vi "lv_icon.vi"(6 "error in (no error)":errorcluster, 7 "VI REF In":refnum<vi>, 8 "From Editor":bool=TRUE, 10 "Color icon in":T8, 11 "BW icon in":T8) -> (0 "Error code out":i32, 2 "Color icon out":T8, 3 "BW icon out":T8, 4 "error out":errorcluster, 5 "VI REF Out":refnum<vi>)   [LabVIEW 2009]
doc: "Version 2.2"
uses:
  <vilib>/picture/picture.llb/imagedata.ctl
  lv_icon_SubVis/Controls/Enum/ENUM_Icon Fixer Commands.ctl
  lv_icon_SubVis/Controls/Enum/ENUM_Graphic Template select.ctl
  lv_icon_SubVis/Controls/Cluster/CLuster_Line Fit Results.ctl
  lv_icon_SubVis/Controls/Enum/ENUM RB_Fit Result.ctl
  lv_icon_SubVis/Controls/String_Picture/Picture_Icon.ctl
  lv_icon_SubVis/Controls/Enum/ENUM_Icon Sizing.ctl
  lv_icon_SubVis/Controls/Enum/RBENUM_Icon Position.ctl
  lv_icon_SubVis/Controls/Cluster/Cluster_Icon Fixer Command Data Set.ctl
  lv_icon_SubVis/Controls/Enum/ENUM_Clear Text Select.ctl
  lv_icon_SubVis/Controls/Enum/ENUM_Set Focus Select.ctl
  lv_icon_SubVis/Controls/Enum/ENUM_Frame Template Select.ctl
  lv_icon_SubVis/Controls/Array/String Array_Body Text.ctl
  lv_icon_SubVis/Controls/String_Picture/STRING_Line Display.ctl
  <vilib>/event_ctls.llb/eventvkey.ctl
  lv_icon_SubVis/Controls/Cluster/Cluster_Sizing Data.ctl
panel:
  in  "stop Keys":bool
  in  "Position":T1=enum."MID-CTR"
  in  "Rule":T2
  in  "Header":bool=TRUE
  in  "Rows":u32=5 min=1 max=5 step=1
  in  "Width":u32=32 min=7 max=32 step=1
  in  "Default sizing":bool
  in  "Random Colors":bool
  out "stop draw":bool
  in  "Reset to Old":bool
  in  "Clear All text":bool
  out "Old":T3 caption="Icon"
  in  "Exit Use Old":bool
  out "New":T3 caption="Icon"
  in  "Exit Use New":bool
  out "History":T3[](array[typedef])
  in  "Frame Select":enum32{"2 Color", "5 Color"}(tab)
  out "Secondary":u32(colorbox)=16448250
  out "Primary":u32(colorbox)=239
  out "Body Back":u32(colorbox)=16448250 caption="Back"
  out "Body txt":u32(colorbox) caption="Text"
  out "Frame":u32(colorbox)
  out "Header txt":u32(colorbox)=65793 caption="Text"
  out "Header Back":u32(colorbox)=239 caption="Back"
  in  "NI Editor":bool
  in  "Close Vi Ref":bool
  out "VI Name":string
  in  "Line 4":string
  in  "Line 3":string
  in  "Line 2":string
  in  "Line 1":string
  in  "Header":string
  out "Data Array":T4[](array[typedef])
  in  "Select Graphic In":T6
  out "Cmd":T7=enum."Initialize"
  out "Big ICON":picture caption="Icon"
  out "timed out?":bool
  # "Icon Sizing"
  # "History"
  # "Make your own icon editor..."
  # "Use this template to create your own icon editor that replaces the built-in LV icon editor. To do so, you must save your new editor as \"lv_icon.vi\" in the same plugins directory where this template resides. Thereafter, whenever you edit an icon in LabVIEW, this VI will execute in place of the LV icon editor. \n\nThe VI's current black/white and color icons are passed as inputs. Your editor should output the modified black/white and color icons and an error code. If you output any non-zero error code, the VI's icons will not be modified. Error code 43 (cancelError) will simply leave the icon unchanged. All other error codes will cause LV's built-in icon editor to launch. This is useful in case there's a bug in your plug-in icon editor.\n\nDo not change connector pane. Do not change the names of any of the  controls or indicators connected to the conpane. You may hide any or all of these controls and add whatever interface you desire. You may decide to call a third party graphics editing tool and leverage that tool for editing your icons in LV."
  # "Body Back\nHeader Text"
  # "Frame\nBody Text\nHeader Back"
  # "Body"
  # "Header"
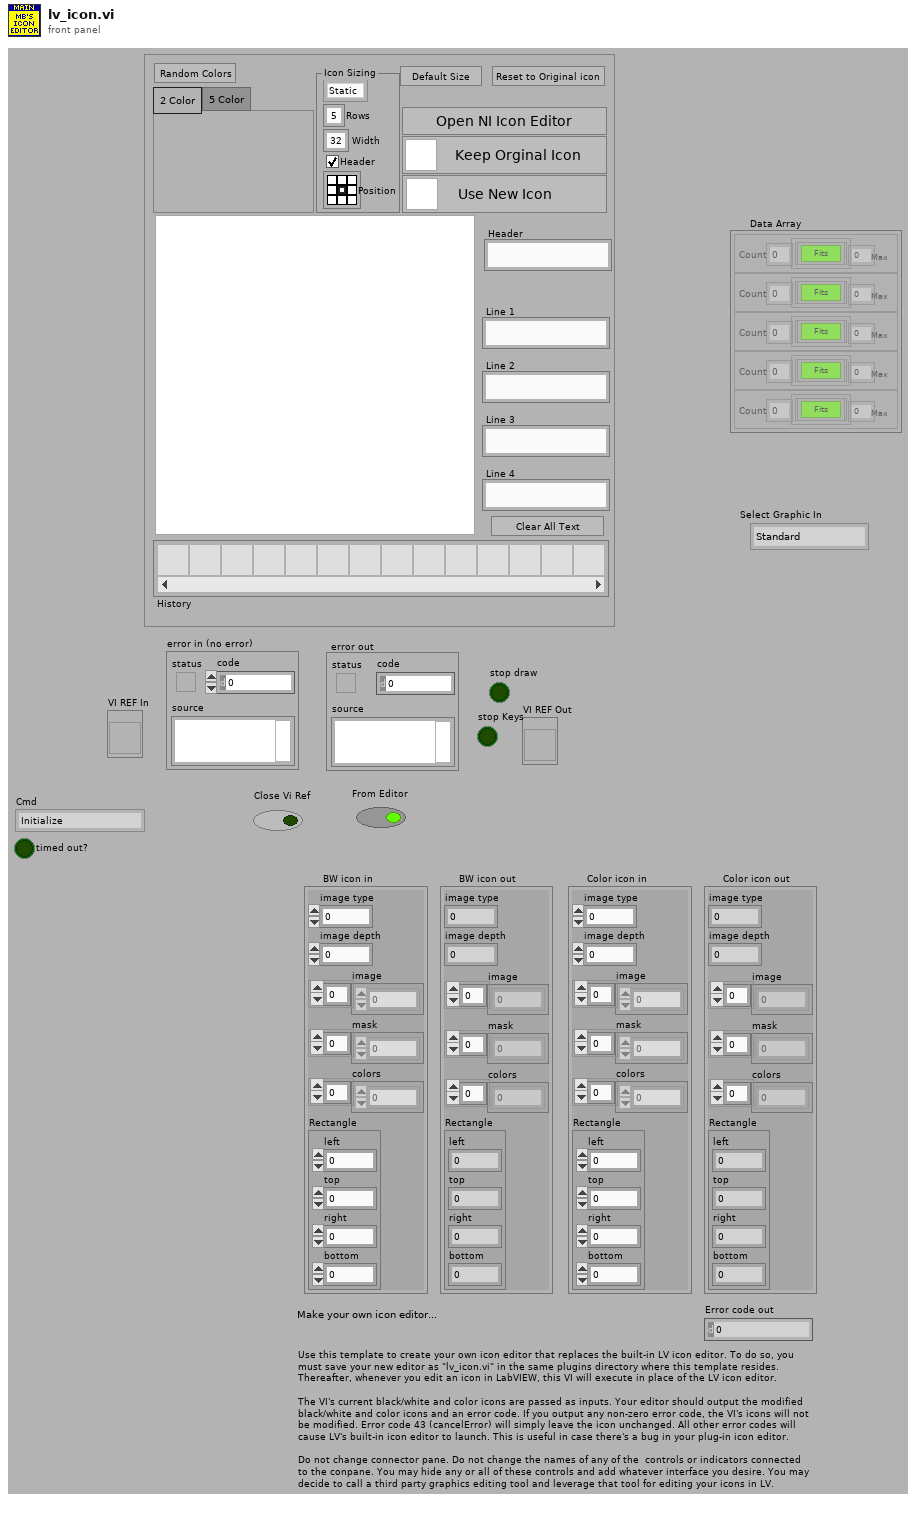
[diagram p1: front panel]
types:
  T1 = typedef "RBENUM_Icon Position.ctl" = enum32{"LFT-TOP", "MID-TOP", "RGT-TOP", "LFT-CTR", "MID-CTR", "RGT-CTR", "LFT-BOT", "MID-BOT", "RGT-BOT"}
  T2 = typedef "ENUM_Icon Sizing.ctl" = enum16{"Static", "Auto"}
  T3 = typedef "Picture_Icon.ctl" = picture
  T4 = typedef "CLuster_Line Fit Results.ctl" = cluster{"Fit Result":T5, "Max":i32, "Count":i32}
  T5 = typedef "ENUM RB_Fit Result.ctl" = enum32{"Fits", "Almost Fits", "NO Fit"}
  T6 = typedef "ENUM_Graphic Template select.ctl" = enum16{"Standard", "Standard Read", "Standard Change", "Auto Test Template"}
  T7 = typedef "ENUM_Icon Fixer Commands.ctl" = enum16{"NoNe", "Initialize", "Get VI", "Extract Icon", "ReDraw New Icon", "Set Vis Icon", "Save Vi", "Clear String controls", "Set Icon Cluster", "Reset Vis Icon", "Pick Colors", "Upload icon templates", "Download icon templates", "Stop Program", "OCR", "Display Set", "Set Focus", "Set Colors"}
  T8 = typedef "imagedata.ctl" = cluster{"image type":i32, "image depth":i32, "image":u8[], "mask":u8[], "colors":u32[], "Rectangle":cluster{"left":i16, "top":i16, "right":i16, "bottom":i16}}
  T9 = typedef "ENUM_Set Focus Select.ctl" = enum16{"NoNe", "Header", "Line 1", "Line 2", "Line 3", "Line 4", "Next", "Back"}
  T10 = typedef "ENUM_Clear Text Select.ctl" = enum16{"NoNe", "All", "Header", "Body"}
  T11 = enum32{"Invalid", "Standard", "Closed", "Hidden", "Minimized", "Maximized"}
  T12 = typedef "Cluster_Icon Fixer Command Data Set.ctl" = cluster{"Cmd":T7, "Data":variant}
  T13 = typedef "Cluster_Icon Data.ctl" = cluster{"Header":T14, "Body":T15, "ImageData":T16, "New Icon":T3, "Line Status":bool[], "Format":T18}
  T14 = typedef "STRING_Line Display.ctl" = string
  T15 = typedef "String Array_Body Text.ctl" = T14[]
  T16 = typedef "Cluster_Image Data.ctl" = cluster{"image type":i32, "image depth":i32, "image":u8[], "mask":u8[], "colors":u32[], "Rectangle":T17}
  T17 = typedef "CLuster_Selectoin Box.ctl" = cluster{"left":i16, "top":i16, "right":i16, "bottom":i16}
  T18 = typedef "Cluster_Icon Format.ctl" = cluster{"Color":T19, "Icon Sizing":T21}
  T19 = typedef "Cluster_Icon Color Set.ctl" = cluster{"Body txt":u32, "Body Back":u32, "Frame":u32, "Header txt":u32, "Header Back":u32, "type":T20}
  T20 = typedef "ENUM_Frame Template Select.ctl" = enum16{"2 Color", "5 Color"}
  T21 = typedef "Cluster_Sizing Data.ctl" = cluster{"Rule":T2, "Header":bool, "Rows":u32, "Width":u32, "Position":T1}
  T22 = typedef "eventvkey.ctl" = enum16{"ASCII", "Enter", "Return", "Shift", "Ctrl", "Alt", "Cmd", "Opt", "Caps", "NumLock", "Clear", "Break", "Up", "Down", "Left", "Right", "Insert", "Delete", "Home", "End", "PageUp", "PageDown", "Escape", "Help", "Pause", "ScrollLock", "F1", "F2", "F3", "F4", "F5", "F6", "F7", "F8", "F9", "F10", "F11", "F12", "F13", "F14", "F15", "F16", "F17", "F18", "F19", "F20", "F21", "F22", "F23", "F24", "Play", "VolumeUp", "VolumeDown", "Mute", "Two Byte Char"}
  T23 = typedef "LVRectTypeDef.ctl" = cluster{"left":i16, "top":i16, "right":i16, "bottom":i16}
  T24 = typedef "LVPoint32TypeDef.ctl" = cluster{"Horizontal":i32, "Vertical":i32}
  T25 = typedef "Bool_Otagon Stop Button no latch.ctl" = bool
  T26 = cluster{"Selection Start":u32, "Selection End":u32}
  T27 = cluster{"Rule":T2, "Header":bool, "Rows":u32, "Width":u32, "Position":T1}
  T28 = typedef "Cluster_Format Storage.ctl" = cluster{"Header":T14, "Format":T18}
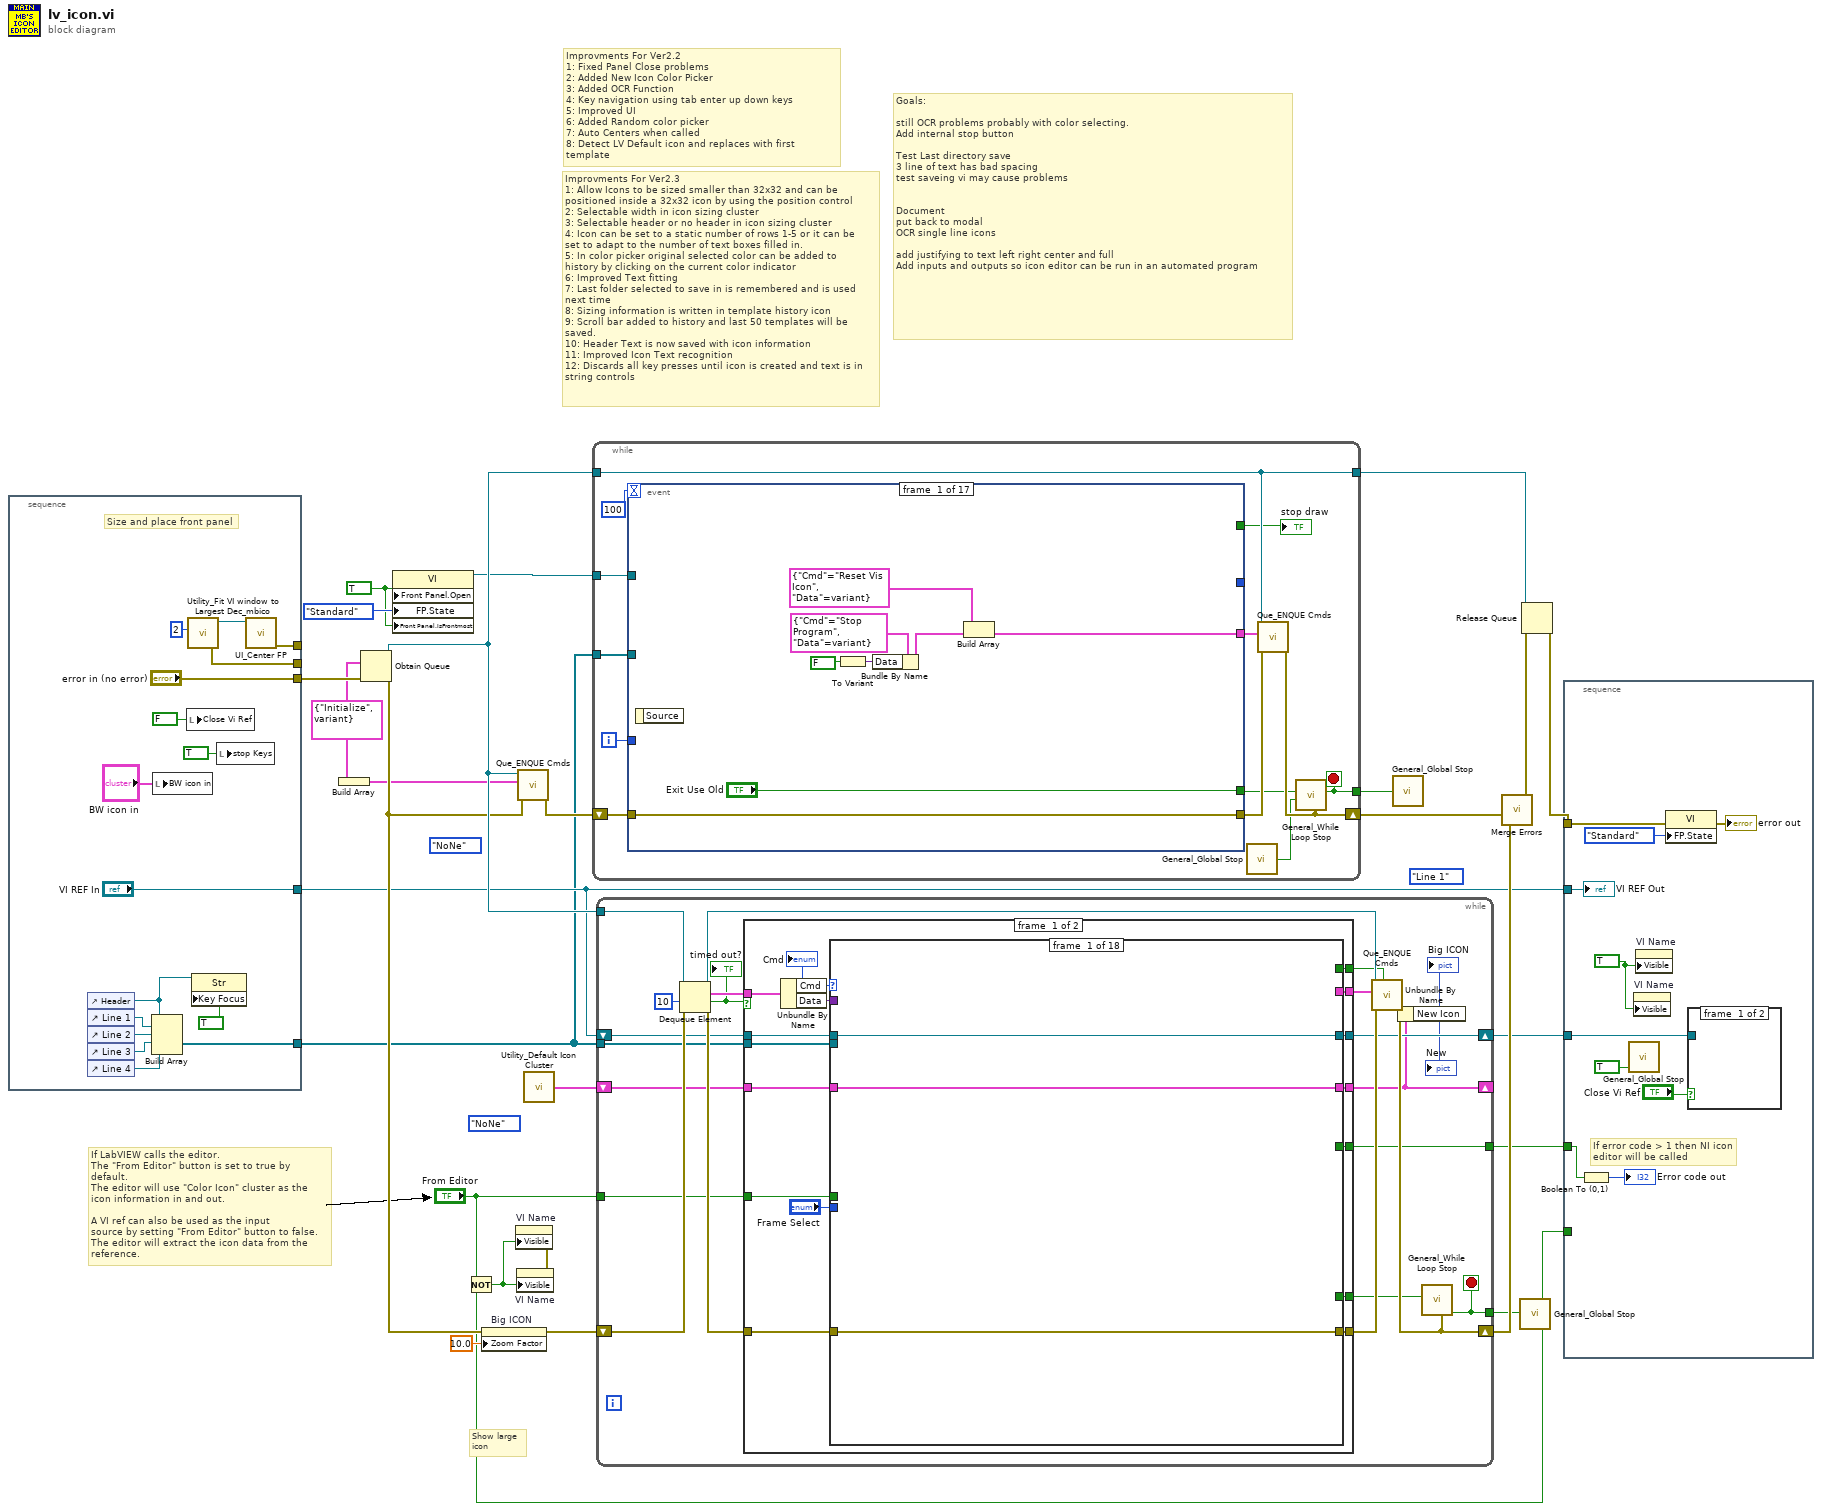
[diagram p0: block diagram]
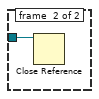
[diagram p2: hidden frame]
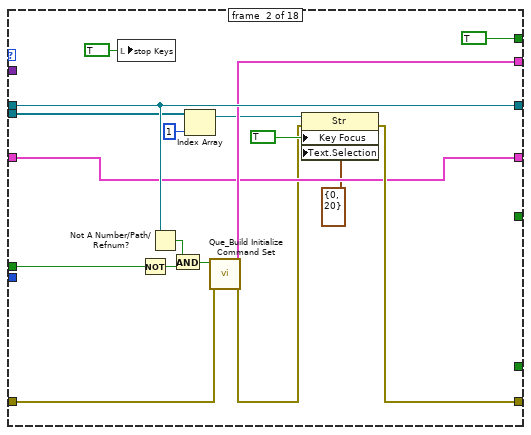
[diagram p3: hidden frame]
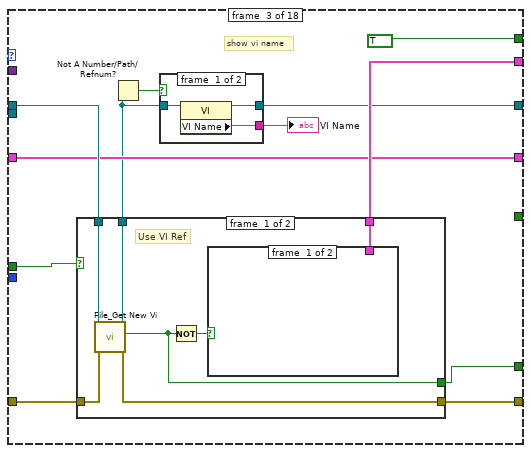
[diagram p4: hidden frame]
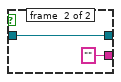
[diagram p5: hidden frame]
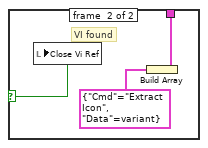
[diagram p6: hidden frame]
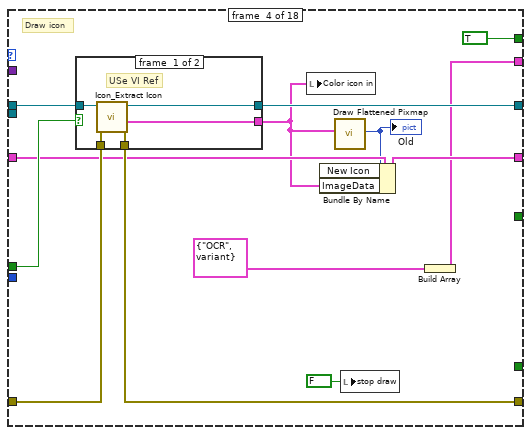
[diagram p8: hidden frame]
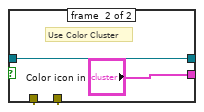
[diagram p9: hidden frame]
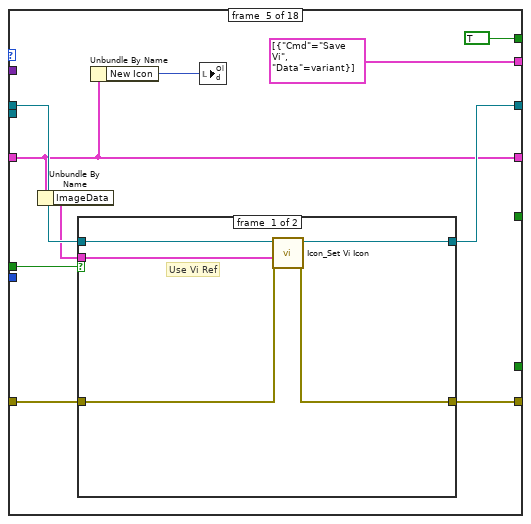
[diagram p10: hidden frame]
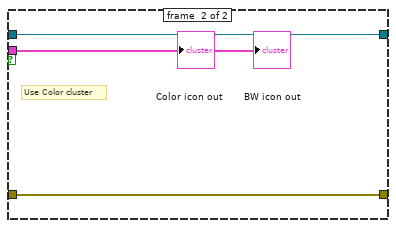
[diagram p11: hidden frame]
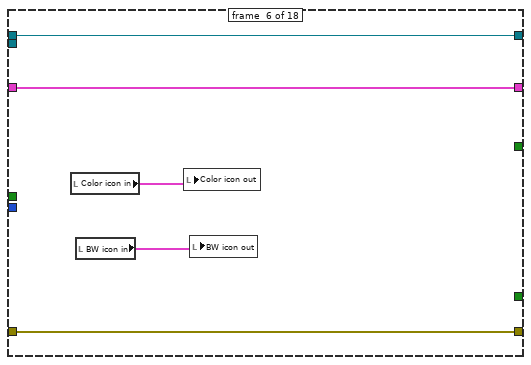
[diagram p12: hidden frame]
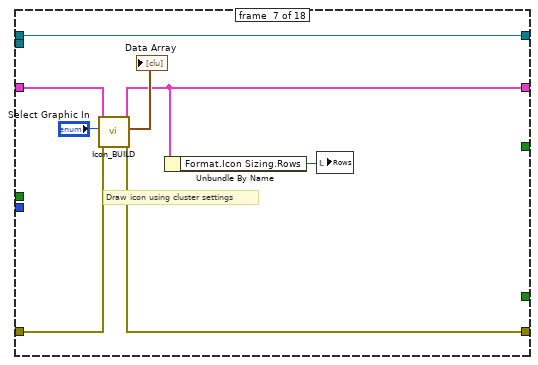
[diagram p13: hidden frame]
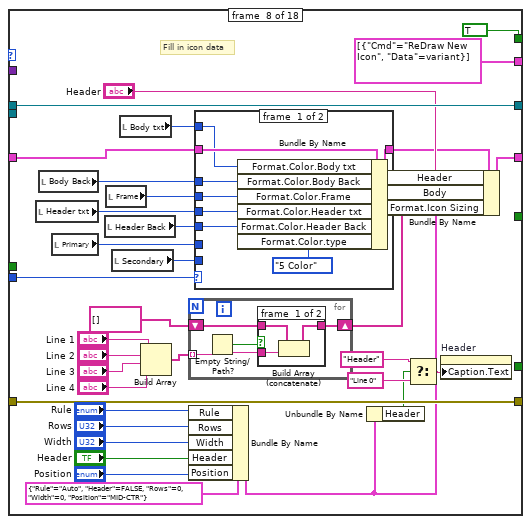
[diagram p14: hidden frame]
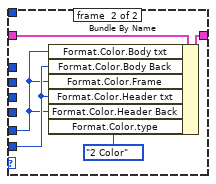
[diagram p16: hidden frame]
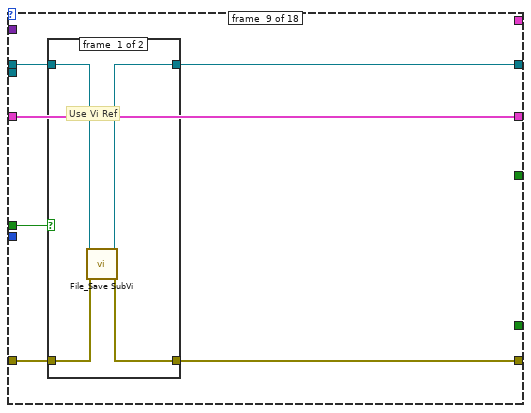
[diagram p17: hidden frame]
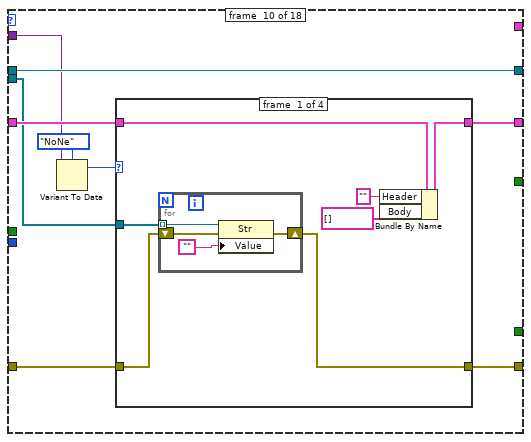
[diagram p19: hidden frame]
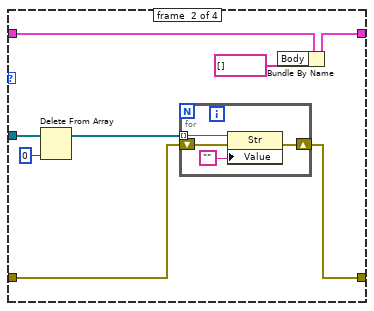
[diagram p20: hidden frame]
diagram:
  (unwired) ENUM_Set_Focus_Select."NoNe" ("Focus Select")
  (unwired) ENUM_Set_Focus_Select."Line 1" ("t")
  (unwired) ENUM_Clear_Text_Select."NoNe" ("Clear Text Select")
  w6 = TRUE ("Front Panel Window:Open")
  w12 = T12 {"Cmd"=enum."Initialize", "Data"=variant} ("Cluster")
  # "Improvments For Ver2.2\n1: Fixed Panel Close problems\n2: Added New Icon Color Picker\n3: Added OCR Function\n4: Key navigation using tab enter up down keys\n5: Improved UI \n6: Added Random color picker\n7: Auto Centers when called\n8: Detect LV Default icon and replaces with first template"
  # "Goals:\n\nstill OCR problems probably with color selecting.\nAdd internal stop button\n\nTest Last directory save\n3 line of text has bad spacing\ntest saveing vi may cause problems\n\n\nDocument\nput back to modal\nOCR single line icons\n \nadd justifying to text left right center and full\nAdd inputs and outputs so icon editor can be run in an automated program"
  # "Improvments For Ver2.3\n1: Allow Icons to be sized smaller than 32x32 and can be \npositioned inside a 32x32 icon by using the position control\n2: Selectable width in icon sizing cluster\n3: Selectable header or no header in icon sizing cluster\n4: Icon can be set to a static number of rows 1-5 or it can be\nset to adapt to the number of text boxes filled in.\n5: In color picker original selected color can be added to \nhistory by clicking on the current color indicator\n6: Improved Text fitting\n7: Last folder selected to save in is remembered and is used \nnext time\n8: Sizing information is written in template history icon\n9: Scroll bar added to history and last 50 templates will be saved.\n10: Header Text is now saved with icon information\n11: Improved Icon Text recognition\n12: Discards all key presses until icon is created and text is in \nstring controls"
  # "Show large\nicon"
  # "If LabVIEW calls the editor.\nThe \"From Editor\" button is set to true by default.\nThe editor will use \"Color Icon\" cluster as the \nicon information in and out.\n\nA VI ref can also be used as the input \nsource by setting \"From Editor\" button to false.\nThe editor will extract the icon data from the \nreference."
  n1 = stacked-sequence {
    tunnel: ["error in (no error)"] -> w22
    tunnel: ["VI REF In"] -> w10
    tunnel: [w37] -> w1
    tunnel: [w28] -> _
    tunnel: [w27] -> _
    frame #0 {
      # "Size and place front panel"
      n2 = control-ref of="Header"() -> (w35:refnum<vi>)
      n3 = control-ref of="Line 1"() -> (w38:refnum<vi>)
      n4 = control-ref of="Line 2"() -> (w39:refnum<vi>)
      n5 = control-ref of="Line 3"() -> (w40:refnum<vi>)
      n6 = control-ref of="Line 4"() -> (w41:refnum<vi>)
      n7 = Build Array(w35, w38, w39, w40, w41) -> (w37:refnum<vi>[])
      n8 = local write "BW icon in"("BW icon in") -> ()
      n9 = local write "Close Vi Ref"(FALSE ("Close Vi Ref")) -> ()
      n10 = call "Utility_Fit VI window to Largest Dec_mbico.vi"("border spacing (2 px)"=2) -> ("error out"=w28:errorcluster, "dup VI Ref"=w32:refnum<vi>)  [unwired: 5 in]
      n11 = property class="Str"(reference=w35, "Key Focus"=TRUE) -> ()  [unwired: 1 in, 2 out]
      n12 = local write "stop Keys"(TRUE ("stop Keys")) -> ()
      n13 = call "UI_Center FP.vi"("VI Ref"=w32) -> ("Error Out"=w27:errorcluster)  [unwired: 9 in, 1 out]
    }
  }
  n14 = Build Array(w12) -> (w11:T12[])
  n15 = Obtain Queue(element data type=w12, error in (no error)=w22) -> (queue out=w21:refnum<queue>, error out=w16:errorcluster)  [unwired: 3 in, 1 out]
  n16 = property class="VI"("Front Panel.Open"=w6, "FP.State"=T11."Standard" ("Front Panel Window:State"), "Front Panel.IsFrontmost"=w6) -> (reference out=w14:refnum<vi>)  [unwired: 2 in, 1 out]
  n17 = Not(x="From Editor") -> (.not. x?=w2:bool)
  n18 = property on="Big ICON" class="Picture"(error in=w16, "Zoom Factor"=sgl 10.0) -> (error out=w15:errorcluster)  [unwired: 1 in, 1 out]
  n19 = property on="VI Name" class="Str"("Visible"=w2) -> (error out=w3:errorcluster)  [unwired: 2 in, 1 out]
  n20 = property on="VI Name" class="Str"(error in=w3, "Visible"=w2) -> ()  [unwired: 1 in, 2 out]
  n21 = call "Que_ENQUE Cmds.vi"("Error"=w16, "Array"=w11, "Queue Ref"=w21) -> ("Error Out"=w20:errorcluster)  [unwired: 8 in]
  n22 = call "Utility_Default Icon Cluster.vi"() -> ("Default Cluster"=w13:T13)  [unwired: 2 in]
  n23 = while {
    shift-right: [w52] -> w25
    shift-left: w20 -> [w48]
    tunnel: w21 -> [w49]
    tunnel: [w49] -> w26
    tunnel: [w50] -> w9
    tunnel: w14 -> [w47]
    tunnel: w1 -> [w43]
    i -> [w45]
    stop <- w50 stop-if-true
    n24 = event shown="[4] \"NI Editor\": Value Change" {
      selector: _ -> [_ _ _ _ _ _ _ _ _ _ _ _ _ _ _ _ _]
      dyn-events: _ -> [_ _ _ _ _ _ _ _ _ _ _ _ _ _ _ _ _]
      timeout: 100 -> [_ _ _ _ _ _ _ _ _ _ _ _ _ _ _ _ _]
      tunnel: w48 -> [w63 w65 w71 w81 w89 w98 w99 w109 w129 w141 w148 w155 w193 w211 w213 w215 w217]
      tunnel: [w63 w65 w71 w81 w89 w98 w99 w110 w129 w133 w148 w154 w192 w211 w213 w215 w217] -> w54
      tunnel: ["Exit Use Old" _ _ "Exit Use New" "NI Editor" TRUE _ _ _ _ _ _ _ _ _ _ _] -> w51
      tunnel: [w62 w66 T12[] [{"Cmd"=enum."Initialize", "Data"=variant}] w80 w88 w90 w101 w107 _ w140 T12[] [{"Cmd"=enum."Set Icon Cluster", "Data"=variant}] w152 w191 T12[] [{"Cmd"=enum."Set Icon Cluster", "Data"=variant}] T12[] [{"Cmd"=enum."ReDraw New Icon", "Data"=variant}] T12[] [{"Cmd"=enum."Set Icon Cluster", "Data"=variant}] w219] -> w53
      tunnel: w47 -> [_ _ _ _ _ _ _ w117 w128 _ _ _ _ _ _ _ _]
      tunnel: w45 -> [_ _ _ _ _ _ _ _ w127 _ _ _ _ _ _ _ _]
      tunnel: [_ _ _ _ _ _ _ _ w124 _ _ _ _ _ _ _ _] -> w44
      tunnel: w43 -> [_ _ _ _ _ _ _ _ _ _ _ w151 w189 _ _ _ _]
      tunnel: [_ _ _ _ _ _ _ _ _ w136 _ _ _ _ _ _ _] -> _
      event #0 {
        n25 = event-data() -> ()  [unwired: 1 in, 1 out]
        n26 = To Variant(anything=FALSE) -> (Variant=w59:variant)
        n27 = Bundle By Name(cluster=T12 {"Cmd"=enum."Stop Program", "Data"=variant} ("element"), "Data"=w59) -> (w60:T12)
        n28 = Build Array(T12 {"Cmd"=enum."Reset Vis Icon", "Data"=variant} ("element"), w60) -> (w62:T12[])
      }
      event #1 {
        n29 = event-data() -> ()  [unwired: 1 in, 1 out]
        n30 = To Variant(anything=ENUM_Clear_Text_Select."All" ("Clear Text Select")) -> (Variant=w67:variant)
        n31 = Bundle By Name(cluster=T12 {"Cmd"=enum."Clear String controls", "Data"=variant} ("Cluster"), "Data"=w67) -> (w69:T12)
        n32 = Build Array(w69, T12 {"Cmd"=enum."ReDraw New Icon", "Data"=variant} ("element")) -> (w66:T12[])
      }
      event #2 {
        n33 = event-data() -> ()  [unwired: 1 in, 1 out]
      }
      event #3 {
        n34 = event-data() -> ()  [unwired: 1 in, 1 out]
        n35 = To Variant(anything=FALSE) -> (Variant=w77:variant)
        n36 = Bundle By Name(cluster=T12 {"Cmd"=enum."Stop Program", "Data"=variant} ("element"), "Data"=w77) -> (w78:T12)
        n37 = Build Array(T12 {"Cmd"=enum."Download icon templates", "Data"=variant} ("element"), T12 {"Cmd"=enum."Set Vis Icon", "Data"=variant} ("element"), w78) -> (w80:T12[])
      }
      event #4 {
        n38 = event-data() -> ()  [unwired: 1 in, 1 out]
        n39 = To Variant(anything=TRUE) -> (Variant=w85:variant)
        n40 = Bundle By Name(cluster=T12 {"Cmd"=enum."Stop Program", "Data"=variant} ("element"), "Data"=w85) -> (w86:T12)
        n41 = Build Array(T12 {"Cmd"=enum."Reset Vis Icon", "Data"=variant} ("element"), w86) -> (w88:T12[])
      }
      event #5 {
        n42 = event-data() -> ()  [unwired: 1 in, 1 out]
        n43 = To Variant(anything=TRUE) -> (Variant=w93:variant)
        n44 = Bundle By Name(cluster=T12 {"Cmd"=enum."Stop Program", "Data"=variant} ("element"), "Data"=w93) -> (w94:T12)
        n45 = Build Array(T12 {"Cmd"=enum."Reset Vis Icon", "Data"=variant} ("element"), w94) -> (w90:T12[])
        n46 = event-data("Discard?"=TRUE) -> ()  [unwired: 1 in, 1 out]
      }
      event #6 {
        n47 = event-data() -> ()  [unwired: 1 in, 1 out]
        n48 = Build Array(T12 {"Cmd"=enum."Set Colors", "Data"=variant} ("element")) -> (w101:T12[])
      }
      event #7 {
        n49 = event-data() -> ("CtlRef"=w116:refnum<vi>)  [unwired: 1 in, 7 out]
        n50 = property class="VI"(reference=w117) -> ("Front Panel.WinBounds"=w115:T23)  [unwired: 1 in, 2 out]
        n51 = property class="ColBox"(reference=w116, error in=w109) -> (reference out=w112:refnum<vi>, error out=w108:errorcluster, "Value"=w114:u32)
        n52 = Unbundle By Name(w115) -> ("left"=w104:i16, "top"=w105:i16)
        n53 = Bundle By Name(cluster=cluster{"Left":i16, "Top":i16} {"Left"=200, "Top"=200} ("Window Origin (0,0) In"), "Left"=w104, "Top"=w105) -> (w103:cluster{"Left":i16, "Top":i16})
        n54 = call "Color Picker_Main.vi"("error in (no error)"=w108, "Window Origin (0,0) In"=w103, "Color In"=w114) -> ("error out"=w111:errorcluster, "Cancled"=w102:bool, "Current Color"=w113:u32)  [unwired: 5 in]
        n55 = case shown="False" w102 {
          tunnel: w113 -> [w122 _]
          tunnel: w112 -> [w121 _]
          tunnel: w111 -> [w120 w123]
          tunnel: [w119 w123] -> w110
          tunnel: [T12[] [{"Cmd"=enum."Set Icon Cluster", "Data"=variant}] _] -> w107
          frame #0 {
            n56 = property class="ColBox"(reference=w121, error in=w120, "Value"=w122) -> (error out=w119:errorcluster)  [unwired: 1 out]
          }
          frame #1 {
          }
        }
      }
      event #8 {
        n57 = event-data() -> ()  [unwired: 1 in, 3 out]
        n58 = Quotient & Remainder(x=w127, y=5) -> (x-y*floor(x/y)=w125:i32)  [unwired: 1 out]
        n59 = case shown="0" w125 {
          tunnel: w128 -> [_ w131]
          frame #0 {
          }
          frame #1 {
            n60 = property class="VI"(reference=w131, "Front Panel.IsFrontmost"=TRUE ("Front Panel Window:Is Frontmost")) -> ()  [unwired: 1 in, 2 out]
          }
        }
        n61 = local read "stop draw"() -> (w124:bool)
      }
      event #9 {
        n62 = event-data() -> ("CtlRef"=w135:refnum<vi>, "Coords"=w134:T24)  [unwired: 1 in]
        n63 = local read "History"() -> (w137:T3[])
        n64 = Array Size(array=w137) -> (size(s)=w136:i32)
        n65 = call "UI_Find Selected History icon.vi"("Border Size"=4, "Error"=w141, "Mouse Cord"=w134, "Array REf"=w135) -> ("Error Out"=w133:errorcluster, "Valid Out"=w132:bool, "Index Out"=w138:i32)  [unwired: 4 in, 1 out]
        n66 = case shown="True" w132 {
          tunnel: [_ w144] -> w140
          tunnel: w138 -> [_ w143]
          frame #0 {
          }
          frame #1 {
            n67 = Increment(x=w143) -> (x+1=w142:i32)
            n68 = To Variant(anything=w142) -> (Variant=w146:variant)
            n69 = Bundle By Name(cluster=T12 {"Cmd"=enum."Pick Colors", "Data"=variant} ("Cluster"), "Data"=w146) -> (w145:T12)
            n70 = Build Array(w145) -> (w144:T12[])
          }
        }
      }
      event #10 {
        n71 = event-data() -> ()  [unwired: 1 in, 1 out]
      }
      event #11 {
        n72 = event-data() -> ("CtlRef"=w156:refnum<vi>, "Char"=w158:i16, "VKey"=w153:T22)  [unwired: 1 in]
        n73 = Build Array(w158) -> (w160:i16[])
        n74 = Byte Array To String(unsigned byte array=w160) -> (string=w159:string)
        n75 = case shown="\"Enter\", \"Return\", \"Up\", \"Down\"" w153 {
          selector: w153 -> [w171 _]
          tunnel: w159 -> [_ w182]
          tunnel: w158 -> [w177 w180]
          tunnel: [w177 w179] -> w157
          tunnel: w156 -> [w170 _]
          tunnel: w155 -> [w169 w178]
          tunnel: [w168 w178] -> w154
          tunnel: [w176 _] -> w152
          tunnel: w151 -> [w166 _]
          frame #0 {
            # "found"
            # "return dey presses"
            n76 = Search 1D Array(1D array=w166, element=w170) -> (index of element=w167:i32)  [unwired: 1 in]
            n77 = Equal?(x=eventvkey."Up", y=w171) -> (x = y?=w164:bool)
            n78 = Select(t=ENUM_Set_Focus_Select."Back" ("Focus Select"), s=w164, f=ENUM_Set_Focus_Select."Next") -> (s? t:f=w161:T9)
            n79 = call "UI_Choose String to set Focus.vi"("Error"=w169, "Current Index"=w167, "Focus Select"=w161, "Ref String  Array"=w166) -> ("Error Out"=w168:errorcluster, "SELECT Out"=w165:T9)  [unwired: 5 in, 1 out]
            n80 = To Variant(anything=w165) -> (Variant=w173:variant)
            n81 = Bundle By Name(cluster=T12 {"Cmd"=enum."Set Focus", "Data"=variant} ("element"), "Data"=w173) -> (w174:T12)
            n82 = Build Array(w174) -> (w176:T12[])
          }
          frame #1 {
            n83 = Printable?(1:w182) -> (0:w181:bool)
            n84 = case shown="True" w181 {
              tunnel: w182 -> [_ w186]
              tunnel: [w183 w184] -> w179
              tunnel: w180 -> [w183 _]
              frame #0 {
              }
              frame #1 {
                # "Capatalize all letters"
                n85 = To Upper Case(1:w186) -> (0:w185:string)
                n86 = String To Byte Array(string=w185) -> (unsigned byte array=w188:u8[])
                n87 = Index Array(array=w188, index=0) -> (element=w184:u8)
              }
            }
          }
        }
        n88 = event-data("Char"=w157, "Discard?"="stop Keys") -> ()  [unwired: 1 in, 1 out]
      }
      event #12 {
        n89 = event-data() -> ("VKey"=w190:T22)  [unwired: 1 in]
        n90 = case shown="Default" w190 {
          selector: w190 -> [w194 _]
          tunnel: w193 -> [w198 w210]
          tunnel: [w197 w210] -> w192
          tunnel: [w199 _] -> w191
          tunnel: w189 -> [w196 _]
          frame #0 {
            n91 = call "UI_Get Focus Index.vi"("Error"=w198, "Ref String  Array"=w196) -> ("Error Out"=w197:errorcluster, "Focus Index Out"=w195:i32)  [unwired: 8 in]
            n92 = case shown="-1" w195 {
              tunnel: [_ w209] -> w199
              tunnel: w194 -> [_ w204]
              frame #0 {
              }
              frame #1 {
                n93 = Equal?(x=eventvkey."Up", y=w204) -> (x = y?=w205:bool)
                n94 = Select(t=ENUM_Set_Focus_Select."Line 4" ("Enum"), s=w205, f=ENUM_Set_Focus_Select."Header" ("Enum")) -> (s? t:f=w200:T9)
                n95 = To Variant(anything=w200) -> (Variant=w206:variant)
                n96 = Bundle By Name(cluster=T12 {"Cmd"=enum."Set Focus", "Data"=variant} ("element"), "Data"=w206) -> (w207:T12)
                n97 = Build Array(w207) -> (w209:T12[])
              }
            }
          }
          frame #1 {
          }
        }
      }
      event #13 {
        n98 = event-data() -> ()  [unwired: 1 in, 1 out]
      }
      event #14 {
        n99 = event-data() -> ()  [unwired: 1 in, 1 out]
      }
      event #15 {
        n100 = event-data() -> ()  [unwired: 1 in, 6 out]
      }
      event #16 {
        n101 = event-data() -> ()  [unwired: 1 in, 6 out]
        n102 = flat-sequence {
          tunnel: [T12[] [{"Cmd"=enum."Set Icon Cluster", "Data"=variant}]] -> w219
          tunnel: T21 {"Rule"=enum."Static", "Header"=TRUE, "Rows"=5, "Width"=32, "Position"=enum."LFT-TOP"} ("Icon Sizing") -> [w225]
          frame #0 {
            n103 = Unbundle By Name(w225) -> ("Rule"=w222:T2, "Header"=w223:bool, "Rows"=w224:u32, "Width"=w221:u32, "Position"=w220:T1)
            n104 = local write "Rule"(w222) -> ()
            n105 = local write "Header"(w223) -> ()
            n106 = local write "Rows"(w224) -> ()
            n107 = local write "Width"(w221) -> ()
            n108 = local write "Position"(w220) -> ()
          }
        }
      }
    }
    "stop draw" <- w44
    n109 = call "General_Global Stop.vi"() -> ("Output"=w46:T25)  [unwired: 5 in]
    n110 = call "Que_ENQUE Cmds.vi"("Error"=w54, "Array"=w53, "Queue Ref"=w49) -> ("Error Out"=w52:errorcluster)  [unwired: 8 in]
    n111 = call "General_While Loop Stop.vi"("Error In"=w52, "Stop 3 In"=w46, "Stop 2 In"=w51) -> ("Stop Out2"=w50:bool)  [unwired: 4 in, 3 out]
  }
  n112 = while {
    tunnel: w21 -> [w247]
    shift-right: [w236] -> w19
    shift-left: w15 -> [w245]
    tunnel: [w242] -> w8
    shift-right: [w230] -> w18
    shift-left: w10 -> [w241]
    tunnel: w1 -> [w234]
    tunnel: "From Editor" -> [w231]
    shift-right: [w227] -> _
    shift-left: w13 -> [w235]
    tunnel: [w229] -> w5
    stop <- w242 stop-if-true
    n113 = Dequeue Element(queue=w247, timeout in ms (-1)=10, error in (no error)=w245) -> (queue out=w239:refnum<queue>, element=w243:T12, timed out?=w240:bool, error out=w244:errorcluster)
    "timed out?" <- w240
    n114 = case shown="False" w240 {
      tunnel: w244 -> [w263 w643]
      tunnel: w243 -> [w262 _]
      tunnel: [w259 w641] -> w232
      tunnel: w241 -> [w258 w642]
      tunnel: [w257 w642] -> w230
      tunnel: [w256 w643] -> w238
      tunnel: [w255 _] -> w237
      tunnel: w235 -> [w254 w640]
      tunnel: [w253 _] -> w233
      tunnel: w234 -> [w252 _]
      tunnel: w231 -> [w251 _]
      tunnel: [w250 w640] -> w227
      tunnel: [w249 _] -> w229
      frame #0 {
        n115 = Unbundle By Name(w262) -> ("Cmd"=w261:T7, "Data"=w260:variant)
        "Cmd" <- w261
        n116 = case shown="\"Upload icon templates\"" w261 {
          tunnel: w263 -> [w264 w268 w295 w322 w338 w354 w362 w396 w425 w440 w480 w513 w526 w531 w548 w551 w608 w635]
          tunnel: [w264 w280 w294 w321 w337 w354 w363 w396 w424 w439 w481 w512 w522 w540 w548 w564 w608 w634] -> w256
          tunnel: w260 -> [_ _ _ _ _ _ _ _ _ w433 w482 _ _ _ w544 _ _ w637]
          tunnel: [_ _ w292 _ _ _ _ _ _ _ _ _ _ _ TRUE _ _ _] -> w259
          tunnel: w258 -> [w266 w283 w293 w324 w343 w352 w364 w398 w423 w438 w484 w518 w528 w541 w546 w565 w609 w638]
          tunnel: [w266 w283 w286 w325 w342 w352 w364 w398 w422 w438 w484 w518 w528 w541 w546 w565 w609 w638] -> w257
          tunnel: [_ w278 w291 w315 T12[] [{"Cmd"=enum."Save Vi", "Data"=variant}] _ _ T12[] [{"Cmd"=enum."ReDraw New Icon", "Data"=variant}] _ _ T12[] [{"Cmd"=enum."Display Set", "Data"=variant}] T12[] [{"Cmd"=enum."Display Set", "Data"=variant}] _ _ _ w559 w607 _] -> w255
          tunnel: w254 -> [w265 w277 w288 w320 w334 w353 w359 w397 w420 w437 w476 w517 w527 w536 w543 w554 w604 w639]
          tunnel: [_ TRUE TRUE TRUE TRUE _ _ TRUE _ _ TRUE TRUE _ _ _ TRUE w606 _] -> w253
          tunnel: w252 -> [_ w279 _ _ _ _ _ _ _ w435 _ _ _ _ _ _ _ w633]
          tunnel: w251 -> [_ w281 w289 w323 w339 _ _ _ w421 _ _ _ _ _ _ _ _ _]
          tunnel: [w265 w277 w288 w319 w334 w353 w358 w387 w420 w436 w475 w519 w527 w536 w543 w561 w604 w639] -> w250
          tunnel: [_ _ _ _ _ _ _ _ _ _ _ _ _ _ w542 _ _ _] -> w249
          tunnel: "Frame Select" -> [_ _ _ _ _ _ _ w376 _ _ _ w511 _ _ _ _ _ _]
          frame #0 {
          }
          frame #1 {
            n117 = local write "stop Keys"(TRUE ("stop Keys")) -> ()
            n118 = Not(x=w281) -> (.not. x?=w275:bool)
            n119 = Not A Number/Path/Refnum?(number/path/refnum=w283) -> (NaN/Path/Refnum?=w276:bool)
            n120 = And(x=w276, y=w275) -> (x .and. y?=w269:bool)
            n121 = Index Array(array=w279, index=1) -> (element=w271:refnum<vi>)
            n122 = call "Que_Build Initialize Command Set.vi"("Error"=w268, "Icon Source Is From A VI"=w269) -> ("Error Out"=w270:errorcluster, "Command Set Out"=w278:T12[])  [unwired: 8 in]
            n123 = property class="Str"(reference=w271, error in=w270, "Key Focus"=TRUE, "Text.Selection"=T26 {"Selection Start"=0, "Selection End"=20}) -> (error out=w280:errorcluster)  [unwired: 1 out]
          }
          frame #2 {
            # "show vi name"
            n124 = case shown="False" w289 {
              tunnel: w295 -> [w307 w312]
              tunnel: [w306 w312] -> w294
              tunnel: w293 -> [w305 w311]
              tunnel: [w304 w311] -> w285
              tunnel: [w303 _] -> w292
              tunnel: [w301 _] -> w291
              frame #0 {
                # "Use VI Ref"
                n125 = call "File_Get New Vi.vi"("VI REF"=w305, "Error"=w307) -> ("VI REF Out"=w304:refnum<vi>, "Vi Not Found Out"=w303:bool, "Error Out"=w306:errorcluster)  [unwired: 6 in]
                n126 = Not(x=w303) -> (.not. x?=w302:bool)
                n127 = case shown="True" w302 {
                  selector: w302 -> [_ w310]
                  tunnel: [_ w308] -> w301
                  frame #0 {
                  }
                  frame #1 {
                    # "VI found"
                    n128 = local write "Close Vi Ref"(w310) -> ()
                    n129 = Build Array(T12 {"Cmd"=enum."Extract Icon", "Data"=variant} ("Cluster")) -> (w308:T12[])
                  }
                }
              }
              frame #1 {
                # "Use Color icon cluster"
              }
            }
            n130 = Not A Number/Path/Refnum?(number/path/refnum=w285) -> (NaN/Path/Refnum?=w284:bool)
            n131 = case shown="False" w284 {
              tunnel: [w298 "" ("Name")] -> w287
              tunnel: w285 -> [w297 w300]
              tunnel: [w296 w300] -> w286
              frame #0 {
                n132 = property class="VI"(reference=w297) -> (reference out=w296:refnum<vi>, "VI Name"=w298:string)  [unwired: 1 in, 1 out]
              }
              frame #1 {
              }
            }
            "VI Name" <- w287
          }
          frame #3 {
            # "Draw icon"
            n133 = case shown="False" w323 {
              tunnel: [w330 w333] -> w325
              tunnel: w324 -> [w329 w333]
              tunnel: w322 -> [w328 w332]
              tunnel: [w327 w332] -> w321
              tunnel: [w326 "Color icon in"] -> w317
              frame #0 {
                # "USe VI Ref"
                n134 = call "Icon_Extract Icon.vi"("VI REF"=w329, "Error"=w328) -> ("VI REF Out"=w330:refnum<vi>, "ImageData Out"=w326:T16, "Error Out"=w327:errorcluster)  [unwired: 6 in]
              }
              frame #1 {
                # "Use Color Cluster"
              }
            }
            n135 = local write "Color icon in"(w317) -> ()
            n136 = call <vilib>:"Draw Flattened Pixmap.vi"("image data"=w317) -> ("new picture"=w318:picture)  [unwired: 8 in]
            "Old" <- w318
            n137 = Bundle By Name(cluster=w320, "New Icon"=w318, "ImageData"=w317) -> (w319:T13)
            n138 = local write "stop draw"(FALSE ("stop draw")) -> ()
            n139 = Build Array(T12 {"Cmd"=enum."OCR", "Data"=variant} ("Cluster")) -> (w315:T12[])
          }
          frame #4 {
            n140 = Unbundle By Name(w334) -> ("ImageData"=w336:T16)
            n141 = case shown="True" w339 {
              tunnel: w343 -> [w348 w351]
              tunnel: [w347 w351] -> w342
              tunnel: w338 -> [w345 w349]
              tunnel: [w344 w349] -> w337
              tunnel: w336 -> [w346 w350]
              frame #0 {
                # "Use Vi Ref"
                n142 = call "Icon_Set Vi Icon.vi"("Error"=w345, "Image Cluster"=w346, "VI REF"=w348) -> ("Error Out"=w344:errorcluster, "VI REF Out"=w347:refnum<vi>)  [unwired: 7 in]
              }
              frame #1 {
                # "Use Color cluster"
                "BW icon out" <- w350
                "Color icon out" <- w350
              }
            }
            n143 = Unbundle By Name(w334) -> ("New Icon"=w335:T3)
            n144 = local write "Old"(w335) -> ()
          }
          frame #5 {
            n145 = local read "Color icon in"() -> (w356:T8)
            n146 = local read "BW icon in"() -> (w355:T8)
            n147 = local write "Color icon out"(w356) -> ()
            n148 = local write "BW icon out"(w355) -> ()
          }
          frame #6 {
            # "Draw icon using cluster settings"
            n149 = call "Icon_BUILD.vi"("Error"=w362, "Select Graphic"="Select Graphic In", "ICON Cluster"=w359) -> ("Error Out"=w363:errorcluster, "Fit Array Out"=→"Data Array":T4[], "ICON Cluster Out"=w358:T13)  [unwired: 6 in]
            n150 = Unbundle By Name(w358) -> ("Format.Icon Sizing.Rows"=w357:u32)
            n151 = local write "Rows"(w357) -> ()
          }
          frame #7 {
            # "Fill in icon data"
            n152 = local read "Header txt"() -> (w382:u32)
            n153 = local read "Body Back"() -> (w379:u32)
            n154 = local read "Primary"() -> (w385:u32)
            n155 = local read "Header Back"() -> (w383:u32)
            n156 = local read "Frame"() -> (w381:u32)
            n157 = local read "Secondary"() -> (w384:u32)
            n158 = local read "Body txt"() -> (w380:u32)
            n159 = Build Array("Line 1", "Line 2", "Line 3", "Line 4") -> (w391:string[])
            n160 = for {
              tunnel: w391 -> [w401] mode=indexing
              shift-right: [w400] -> w388
              shift-left: string[] [] -> [w399]
              n161 = Empty String/Path?(string/path=w401) -> (empty?=w402:bool)
              n162 = case shown="False" w402 {
                tunnel: w401 -> [w404 _]
                tunnel: w399 -> [w405 w406]
                tunnel: [w403 w406] -> w400
                frame #0 {
                  n163 = Build Array (concatenate)(w405, w404) -> (w403:string[])
                }
                frame #1 {
                }
              }
            }
            n164 = Bundle By Name(cluster=T27 {"Rule"=enum."Auto", "Header"=FALSE, "Rows"=0, "Width"=0, "Position"=enum."MID-CTR"} ("Icon Sizing"), "Rule"="Rule", "Rows"="Rows", "Width"="Width", "Header"="Header", "Position"="Position") -> (w370:T27)
            n165 = case shown="\"2 Color\"" w376 {
              tunnel: w397 -> [w411 w419]
              tunnel: w381 -> [w414 _]
              tunnel: w382 -> [w413 _]
              tunnel: w383 -> [w412 _]
              tunnel: w385 -> [_ w415]
              tunnel: w384 -> [_ w416]
              tunnel: [w410 w418] -> w386
              tunnel: w380 -> [w409 _]
              tunnel: w379 -> [w408 _]
              frame #0 {
                n166 = Bundle By Name(cluster=w411, "Format.Color.Body txt"=w409, "Format.Color.Body Back"=w408, "Format.Color.Frame"=w414, "Format.Color.Header txt"=w413, "Format.Color.Header Back"=w412, "Format.Color.type"=ENUM_Frame_Template_Select."5 Color" ("Frame")) -> (w410:T13)
              }
              frame #1 {
                n167 = Bundle By Name(cluster=w419, "Format.Color.Body txt"=w415, "Format.Color.Body Back"=w416, "Format.Color.Frame"=w415, "Format.Color.Header txt"=w416, "Format.Color.Header Back"=w415, "Format.Color.type"=ENUM_Frame_Template_Select."2 Color" ("Frame")) -> (w418:T13)
              }
            }
            n168 = Unbundle By Name(w370) -> ("Header"=w372:bool)
            n169 = Bundle By Name(cluster=w386, "Header"="Header", "Body"=w388, "Format.Icon Sizing"=w370) -> (w387:T13)
            n170 = Select(t="Header" ("Caption.Text"), s=w372, f="Line 0") -> (s? t:f=w374:string)
            n171 = property on="Header" class="Str"("Caption.Text"=w374) -> ()  [unwired: 2 in, 2 out]
          }
          frame #8 {
            n172 = case shown="False" w421 {
              tunnel: w425 -> [w429 w430]
              tunnel: [w428 w430] -> w424
              tunnel: w423 -> [w427 w431]
              tunnel: [w426 w431] -> w422
              frame #0 {
                # "Use Vi Ref"
                n173 = call "File_Save SubVi.vi"("Error"=w429, "VI Ref"=w427) -> ("Error Out"=w428:errorcluster, "VI Ref Out"=w426:refnum<vi>)  [unwired: 8 in]
              }
              frame #1 {
                # "Use color cluster"
              }
            }
          }
          frame #9 {
            n174 = Variant To Data(Variant=w433, type=ENUM_Clear_Text_Select."NoNe" ("Clear Text Select")) -> (data=w432:T10)  [unwired: 1 in, 1 out]
            n175 = case shown="\"All\"" w432 {
              tunnel: w440 -> [w447 w459 w465 w474]
              tunnel: [w446 w458 w465 w473] -> w439
              tunnel: w437 -> [w445 w457 w464 w472]
              tunnel: [w444 w456 w464 w471] -> w436
              tunnel: w435 -> [w441 w454 _ w469]
              frame #0 {
                n176 = for {
                  tunnel: w441 -> [w451] mode=indexing
                  shift-right: [w449] -> w446
                  shift-left: w447 -> [w450]
                  n177 = property class="Str"(reference=w451, error in=w450, "Value"="") -> (error out=w449:errorcluster)  [unwired: 1 out]
                }
                n178 = Bundle By Name(cluster=w445, "Header"=T14 "", "Body"=T15 []) -> (w444:T13)
              }
              frame #1 {
                n179 = Delete From Array(array=w454, index=0) -> (array with subset deleted=w453:refnum<vi>[])  [unwired: 1 in, 1 out]
                n180 = for {
                  tunnel: w453 -> [w463] mode=indexing
                  shift-right: [w461] -> w458
                  shift-left: w459 -> [w462]
                  n181 = property class="Str"(reference=w463, error in=w462, "Value"="") -> (error out=w461:errorcluster)  [unwired: 1 out]
                }
                n182 = Bundle By Name(cluster=w457, "Body"=T15 []) -> (w456:T13)
              }
              frame #2 {
              }
              frame #3 {
                n183 = Index Array(array=w469, index=0) -> (element=w467:refnum<vi>)
                n184 = property class="Str"(reference=w467, error in=w474, "Value"="") -> (error out=w473:errorcluster)  [unwired: 1 out]
                n185 = Bundle By Name(cluster=w472, "Header"=T14 "") -> (w471:T13)
              }
            }
          }
          frame #10 {
            n186 = Variant To Data(Variant=w482, type=0) -> (data=w479:i32)  [unwired: 1 in, 1 out]
            n187 = case shown="1.." w479 {
              selector: w479 -> [w493 _]
              tunnel: w476 -> [w490 _]
              tunnel: [w494 w510] -> w481
              tunnel: w480 -> [w495 w510]
              tunnel: w476 -> [w489 w509]
              tunnel: [w488 w509] -> w475
              frame #0 {
                n188 = Current VI's Path() -> (path=w496:path)
                n189 = call "File_Read Write Icon Template colors.vi"("Read(f)\nWrite(t)"=FALSE ("Read(f)\nWrite(t)"), "Error"=w495, "Home Path"=w496) -> ("Error Out"=w494:errorcluster, "Template Select Out"=w492:T28[])  [unwired: 6 in, 1 out]
                n190 = Array Size(array=w492) -> (size(s)=w491:i32)
                n191 = case shown="1.." w491 {
                  tunnel: w493 -> [_ w508]
                  tunnel: [w499 w506] -> w486
                  tunnel: [w500 w505] -> w487
                  tunnel: w492 -> [_ w504]
                  tunnel: w490 -> [w501 _]
                  tunnel: [w498 w502] -> w485
                  frame #0 {
                    n192 = Unbundle By Name(w501) -> ("Format.Icon Sizing"=w500:T21, "Format.Color"=w499:T19, "Header"=w498:T14)
                  }
                  frame #1 {
                    n193 = Decrement(x=w508) -> (x-1=w503:i32)
                    n194 = Index Array(array=w504, index=w503) -> (element=w507:T28)
                    n195 = Unbundle By Name(w507) -> ("Format.Icon Sizing"=w505:T21, "Format.Color"=w506:T19, "Header"=w502:T14)
                  }
                }
                n196 = Bundle By Name(cluster=w489, "Format.Icon Sizing"=w487, "Format.Color"=w486, "Header"=w485) -> (w488:T13)
              }
              frame #1 {
              }
            }
          }
          frame #11 {
            n197 = call "Icon_Create Random Colors.vi"("Error"=w513, "Frame Select"=w511) -> ("Error Out"=w512:errorcluster, "Color Out"=w514:T19)  [unwired: 8 in]
            n198 = Bundle By Name(cluster=w517, "Format.Color"=w514) -> (w519:T13)
          }
          frame #12 {
            # "Get color sets from file and convert to template Icons"
            n199 = Current VI's Path() -> (path=w521:path)
            n200 = call "File_Read Write Icon Template colors.vi"("Read(f)\nWrite(t)"=FALSE ("Read(f)\nWrite(t)"), "Error"=w526, "Home Path"=w521) -> ("Error Out"=w523:errorcluster, "Template Select Out"=w524:T28[])  [unwired: 6 in, 1 out]
            n201 = call "Icon_Build Template array.vi"("Error"=w523, "Set Array"=w524) -> ("Error Out"=w522:errorcluster, "Template Array Out"=→"History":T3[])  [unwired: 8 in]
          }
          frame #13 {
            # "Add new icon color set to array and save to file"
            n202 = Unbundle By Name(w536) -> ("Header"=w529:T14, "Format"=w535:T18)
            n203 = Current VI's Path() -> (path=w532:path)
            n204 = call "File_Read Write Icon Template colors.vi"("Read(f)\nWrite(t)"=FALSE ("Read(f)\nWrite(t)"), "Error"=w531, "Home Path"=w532) -> ("Error Out"=w530:errorcluster, "Template Select Out"=w533:T28[])  [unwired: 6 in, 1 out]
            n205 = call "Icon_Update Template icon array.vi"("Error"=w530, "Format"=w535, "Header"=w529, "Template Array"=w533) -> ("Error Out"=w538:errorcluster, "Template Array Out"=w537:T28[])  [unwired: 6 in]
            n206 = call "File_Read Write Icon Template colors.vi"("Read(f)\nWrite(t)"=TRUE ("Read(f)\nWrite(t)"), "Error"=w538, "Home Path"=w532, "Template Select"=w537) -> ("Error Out"=w540:errorcluster)  [unwired: 5 in, 2 out]
          }
          frame #14 {
            # "Call NI icon editor"
            n207 = Variant To Data(Variant=w544, type=FALSE) -> (data=w542:bool)  [unwired: 1 in, 1 out]
          }
          frame #15 {
            n208 = Unbundle By Name(w554) -> ("ImageData"=w553:T16)
            n209 = call "Icon_Detect NI Template.vi"("Error"=w551, "Color 256"=w553) -> ("Error Out"=w550:errorcluster, "NI Template Out"=w552:bool)  [unwired: 7 in, 1 out]
            n210 = case shown="False" w552 {
              tunnel: w554 -> [w578 w586]
              tunnel: w550 -> [w577 w583]
              tunnel: [w576 w583] -> w564
              tunnel: [w575 FALSE] -> w562
              tunnel: [w573 w586] -> w561
              tunnel: [w567 ENUM_Set_Focus_Select."Header" ("Enum")] -> w555
              tunnel: [T12 {"Cmd"=enum."NoNe", "Data"=variant} ("Cluster") w581] -> w549
              frame #0 {
                n211 = call "OCR_OCR MAIN.vi"("Error"=w577, "ICON Cluster"=w578) -> ("Error Out"=w576:errorcluster, "ICON Cluster Out"=w573:T13)  [unwired: 8 in]
                n212 = Unbundle By Name(w573) -> ("Line Status"=w572:bool[])
                n213 = And Array Elements(Boolean array=w572) -> (logical AND=w574:bool)
                n214 = Index Array(array=w572, index=0) -> (element=w570:bool)
                n215 = Not(x=w574) -> (.not. x?=w575:bool)
                n216 = Select(t=ENUM_Set_Focus_Select."Line 1", s=w570, f=ENUM_Set_Focus_Select."Header" ("Enum")) -> (s? t:f=w567:T9)
              }
              frame #1 {
                n217 = To Variant(anything=1) -> (Variant=w579:variant)
                n218 = Bundle By Name(cluster=T12 {"Cmd"=enum."Pick Colors", "Data"=variant} ("Cluster"), "Data"=w579) -> (w581:T12)
              }
            }
            n219 = To Variant(anything=w555) -> (Variant=w556:variant)
            n220 = local write "stop draw"(w562) -> ()
            n221 = Bundle By Name(cluster=T12 {"Cmd"=enum."Set Focus", "Data"=variant} ("element"), "Data"=w556) -> (w557:T12)
            n222 = Build Array(T12 {"Cmd"=enum."Display Set", "Data"=variant} ("Cluster"), w557, w549) -> (w559:T12[])
          }
          frame #16 {
            n223 = Unbundle By Name(w604) -> ("Format.Color.type"=w611:T20, "Format.Color.Body txt"=→"Primary" →"Body txt":u32, "Format.Color.Body Back"=→"Secondary" →"Body Back":u32, "Format.Color.Frame"=→"Frame":u32, "Format.Color.Header txt"=→"Header txt":u32, "Format.Color.Header Back"=→"Header Back":u32)
            n224 = Unbundle By Name(w604) -> ("Header"=w598:T14, "Body"=w599:T15)
            n225 = Unbundle By Name(w604) -> ("Format.Icon Sizing"=w588:T21, "Format.Icon Sizing.Header"=w601:bool)
            n226 = local write "Header"(w598) -> ()
            n227 = Index Array(array=w599, index #1=0 ("index"), index #2=1 ("index"), index #3=2 ("index"), index #4=3 ("index")) -> (element #1=w620:T14, element #2=w619:T14, element #3=w618:T14, element #4=w617:T14)
            n228 = local write "Line 1"(w620) -> ()
            n229 = local write "Line 2"(w619) -> ()
            n230 = local write "Line 3"(w618) -> ()
            n231 = local write "Line 4"(w617) -> ()
            n232 = Empty String/Path?(string/path=w598) -> (empty?=w597:bool)
            n233 = To Unsigned Long Integer(number=w611) -> (unsigned 32bit integer=w610:u32)
            n234 = Select(t=ENUM_Set_Focus_Select."Header" ("Focus Select"), s=w597, f=ENUM_Set_Focus_Select."Line 1" ("Focus Select")) -> (s? t:f=w594:T9)
            n235 = local write "Frame Select"(w610) -> ()
            n236 = local read "stop draw"() -> (w605:bool)
            n237 = Select(t="Header" ("Caption.Text"), s=w601, f="Line 0") -> (s? t:f=w602:string)
            n238 = property on="Header" class="Str"("Caption.Text"=w602) -> ()  [unwired: 2 in, 2 out]
            n239 = case shown="False" w605 {
              tunnel: [w625 _] -> w607
              tunnel: [TRUE _] -> w606
              tunnel: w594 -> [w629 _]
              frame #0 {
                n240 = To Variant(anything=w629) -> (Variant=w628:variant)
                n241 = Bundle By Name(cluster=T12 {"Cmd"=enum."Set Focus", "Data"=variant} ("Cluster"), "Data"=w628) -> (w627:T12)
                n242 = Build Array(T12 {"Cmd"=enum."ReDraw New Icon", "Data"=variant} ("Cluster"), w627) -> (w625:T12[])
              }
              frame #1 {
              }
            }
            n243 = Unbundle By Name(w588) -> ("Rule"=w591:T2, "Header"=w592:bool, "Rows"=w593:u32, "Width"=w590:u32, "Position"=w589:T1)
            n244 = local write "stop Keys"(FALSE ("stop Keys")) -> ()
            n245 = local write "Rule"(w591) -> ()
            n246 = local write "Header"(w592) -> ()
            n247 = local write "Rows"(w593) -> ()
            n248 = local write "Width"(w590) -> ()
            n249 = local write "Position"(w589) -> ()
          }
          frame #17 {
            n250 = Variant To Data(Variant=w637, type=ENUM_Set_Focus_Select."NoNe" ("Enum")) -> (data=w632:T9)  [unwired: 1 in, 1 out]
            n251 = call "UI_Set Focus.vi"("Error"=w635, "Focus Select"=w632, "Ref String  Array"=w633) -> ("Error Out"=w634:errorcluster)  [unwired: 8 in]
          }
        }
      }
      frame #1 {
        # "No Commands"
        n252 = call "General_Global Stop.vi"() -> ("Output"=w641:T25)  [unwired: 5 in]
        n253 = case shown="False" w641 {
          frame #0 {
            n254 = Wait Until Next ms Multiple(millisecond multiple=u32 50) -> ()  [unwired: 1 out]
          }
          frame #1 {
          }
        }
      }
    }
    n255 = call "Que_ENQUE Cmds.vi"("Add To Begining"=w233, "Error"=w238, "Array"=w237, "Queue Ref"=w239) -> ("Error Out"=w236:errorcluster)  [unwired: 7 in]
    n256 = Unbundle By Name(w227) -> ("New Icon"=→"Big ICON" →"New":T3)
    n257 = call "General_While Loop Stop.vi"("Error In"=w236, "Stop 2 In"=w232) -> ("Stop Out3"=w242:bool)  [unwired: 5 in, 3 out]
  }
  n258 = call "General_Global Stop.vi"("Set"=w9) -> ()  [unwired: 4 in, 1 out]
  n259 = call <vilib>:"Merge Errors.vi"("error in 3 (no error)"=w25, "error in 2 (no error)"=w19) -> ("error out"=w24:errorcluster)  [unwired: 5 in]
  n260 = call "General_Global Stop.vi"("Set"=w8) -> ()  [unwired: 4 in, 1 out]
  n261 = Release Queue(queue=w26, error in (no error)=w24) -> (error out=w23:errorcluster)  [unwired: 1 in, 2 out]
  n262 = stacked-sequence {
    tunnel: w23 -> [w649]
    tunnel: w18 -> [w653]
    tunnel: w10 -> [w652]
    tunnel: w5 -> [w646]
    tunnel: "From Editor" -> [_]
    frame #0 {
      w645 = TRUE ("Visible")
      # "If error code > 1 then NI icon\neditor will be called"
      n263 = Boolean To (0,1)(Boolean=w646) -> (0, 1=→"Error code out":i16)
      n264 = call "General_Global Stop.vi"("Complete"=TRUE ("reset")) -> ()  [unwired: 4 in, 1 out]
      n265 = property on="VI Name" class="Str"("Visible"=w645) -> ()  [unwired: 2 in, 2 out]
      n266 = property on="VI Name" class="Str"("Visible"=w645) -> ()  [unwired: 2 in, 2 out]
      n267 = property class="VI"(error in=w649, "FP.State"=T11."Standard" ("Front Panel Window:State")) -> (error out=→"error out":errorcluster)  [unwired: 1 in, 1 out]
      n268 = case shown="False" "Close Vi Ref" {
        tunnel: w653 -> [_ w655]
        frame #0 {
        }
        frame #1 {
          n269 = Close Reference(reference=w655) -> ()  [unwired: 1 in, 1 out]
        }
      }
      "VI REF Out" <- w652
    }
  }
